vi "Read IRuleFileParser.vi"(11 "CDependencyInspection in":refnum<class "CDependencyInspection.lvclass">) -> (1 "IRuleFileParser":refnum<class "IRuleFileParser.lvclass">, 3 "CDependencyInspection out":refnum<class "CDependencyInspection.lvclass">)   [LabVIEW 2020, in "DependencyInspection.lvlib" / "CDependencyInspection.lvclass"]
uses:
  CDependencyInspection.lvclass
  obj/Addons/ExtensionInterfaces.lvlibp/IRuleFileParser/IRuleFileParser.lvclass
  CDependencyInspection.lvclass/CDependencyInspection.ctl
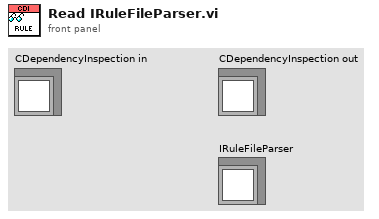
[diagram p1: front panel]
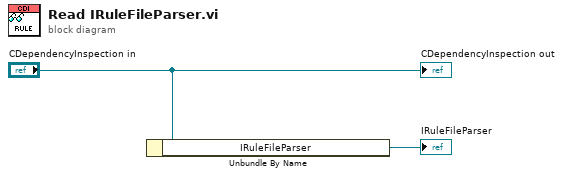
[diagram p0: block diagram]
diagram:
  n1 = Unbundle By Name("CDependencyInspection in") -> ("IRuleFileParser"=→"IRuleFileParser":refnum<class "IRuleFileParser.lvclass">)
  "CDependencyInspection out" <- "CDependencyInspection in"
